vi "SP Convert Display Data.vi"(7 "Old Formatted Data":bool, 10 "Old Data Display":u16(ring) caption="Old Display Data" items=["Data", "Memory", "Data/Memory"]) -> (2 "New Data Display":T1 caption="Data" items=["Data", "Memory", "Data/Memory"], 5 "New Formatted Data":bool)   [LabVIEW 2011]
uses:
  TypeDefs/SP Display Data.ctl
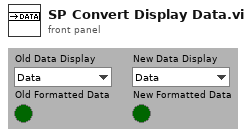
[diagram p1: front panel]
types:
  T1 = typedef "SP Display Data.ctl" = u16
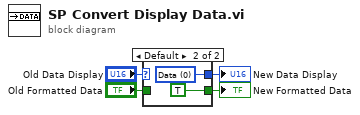
[diagram p0: block diagram]
diagram:
  n1 = case shown="Default" "Old Data Display" {
    selector: "Old Data Display" -> [w6 _]
    tunnel: [w6 w8] -> w1
    tunnel: [w5 TRUE ("Old Formatted Data")] -> w2
    tunnel: "Old Formatted Data" -> [w5 _]
    frame 0 {
    }
    frame Default {
      w8 = T1 0 items=["Data", "Memory", "Data/Memory"] ("New Data Display")
    }
  }
  "New Formatted Data" <- w2
  "New Data Display" <- w1
